vi "HFRR ADV v01.vi"() -> ()   [LabVIEW 2023] (continued)
                n1196 = local write "OK Button 16"(FALSE ("Print 3")) -> ()
              }
            }
          }
        }
        n1197 = case shown="True" "OK Button 17" {
          frame False {
          }
          frame True {
            (unwired) 0  # existing file
            w2745 = "Choose a datalog file to open"  # prompt
            n1198 = local read "String"() -> (w2740:string)
            n1199 = local write "OK Button 17"(FALSE ("OK Button 17")) -> ()
            n1200 = String To Path(string=w2740) -> (path=w2741:path)
            n1201 = File Dialog(6:"*.duf" ("pattern"), 7:w2745, 11:w2741) -> (0:w2732:errorcluster, 3:w2751:path)  [unwired: 4 in, 2 out]
            n1202 = Unbundle(w2732) -> ()  [unwired: 3 out]
            n1203 = Open/Create/Replace File "Open File"(file path (use dialog)=w2751) -> (refnum out=w2743:refnum<file>)  [unwired: 5 in, 2 out]
            n1204 = Path To String(path=w2751) -> (string=w2734:string)
            n1205 = while {
              tunnel: w2743 -> [w2755]
              i -> [w2752]
              stop <- w2753 continue-if-true
              (unwired) TRUE ("line mode (F)")
              n1206 = local write "Numeric 16"(w2752) -> ()
              n1207 = Read from Text File "Read File"(file (use dialog)=w2755) -> (text=w2754:string)  [unwired: 3 in, 3 out]
              n1208 = String Length(string=w2754) -> (length=w2757:i32)
              n1209 = Greater?(x=w2757, y=1) -> (0:w2753:bool)
            }
            n1210 = local write "String 29"(w2734) -> ()
            n1211 = Match Pattern(string=w2734, regular expression=".dwm" ("substring (\"\")")) -> (before substring=w2735:string)  [unwired: 1 in, 3 out]
            "String Indicator 3" <- w2735
            n1212 = Search and Replace String(input string=w2734, search string=".duf", replace string=".dgf" ("replace string (\"\")")) -> (result string=→"String Indicator 4":string)  [unwired: 5 in, 3 out]
            n1213 = String To Path(string=w2735) -> (path=w2742:path)
            "path" <- w2742
            n1214 = Strip Path(path=w2751) -> (name=w2749:string)  [unwired: 1 out]
            n1215 = call <vilib>:"Read Characters From File.vi"("file path (dialog if empty)"=w2742, "start of read offset (chars.:0)"=60 ("start of read offset (chars.: 0)")) -> ("character string"=→"String Indicator 2":string)  [unwired: 4 in, 3 out]
            n1216 = Match Pattern(string=w2749, regular expression=".dwm") -> (before substring=w2733:string)  [unwired: 1 in, 3 out]
            "String Indicator" <- w2733
            n1217 = local write "TITTLE 2"(w2733) -> ()
          }
        }
      }
    }
    n1218 = local read "OK Button 16"() -> (w788:bool)
    n1219 = Or(x=w788, y="OPEN") -> (x .or. y?=w789:bool)
    n1220 = case shown="True" w789 {
      tunnel: w788 -> [_ w841]
      frame False {
      }
      frame True {
        n1221 = stacked-sequence {
          tunnel: w841 -> [_ w908 _ _]
          frame #0 {
            w857 = "  " ("String 6")
            n1222 = local write "OPEN"(FALSE ("open")) -> ()
            n1223 = property on="OPEN" class="Bool (strict)"("Visible"=FALSE) -> ()  [unwired: 2 in, 2 out]
            n1224 = local write "String 12"(w857) -> ()
            n1225 = local write "String 6"(w857) -> ()
            n1226 = local write "String 7"(w857) -> ()
            n1227 = local write "String 8"(w857) -> ()
            n1228 = local read "OK Button 16"() -> (w842:bool)
            n1229 = case shown="True" w842 {
              tunnel: [w858 w859] -> w846
              frame False {
                n1230 = local read "string1"() -> (w858:string)
              }
              frame True {
                n1231 = local read "String Indicator 4"() -> (w859:string)
              }
            }
            n1232 = local read "string1 2"() -> (w845:string)
            n1233 = local read "string1 4"() -> (w843:string)
            n1234 = local read "string1 3"() -> (w844:string)
            n1235 = String To Path(string=w846) -> (path=w854:path)
            n1236 = String To Path(string=w845) -> (path=w853:path)
            n1237 = String To Path(string=w844) -> (path=w852:path)
            n1238 = String To Path(string=w843) -> (path=w851:path)
            n1239 = Open/Create/Replace File "Open File"(file path (use dialog)=w854) -> (refnum out=w850:refnum<file>)  [unwired: 5 in, 2 out]
            n1240 = Open/Create/Replace File "Open File"(file path (use dialog)=w853) -> (refnum out=w849:refnum<file>)  [unwired: 5 in, 2 out]
            n1241 = Open/Create/Replace File "Open File"(file path (use dialog)=w852) -> (refnum out=w848:refnum<file>)  [unwired: 5 in, 2 out]
            n1242 = Open/Create/Replace File "Open File"(file path (use dialog)=w851) -> (refnum out=w847:refnum<file>)  [unwired: 5 in, 2 out]
            n1243 = while {
              tunnel: w850 -> [w865]
              i -> [w861]
              stop <- w860 continue-if-true
              (unwired) TRUE ("line mode (F)")
              n1244 = Read from Text File "Read File"(file (use dialog)=w865) -> (text=w862:string)  [unwired: 3 in, 3 out]
              n1245 = local write "Numeric 8"(w861) -> ()
              n1246 = String Length(string=w862) -> (length=w864:i32)
              n1247 = Greater?(x=w864, y=1) -> (0:w860:bool)
            }
            n1248 = while {
              tunnel: w849 -> [w871]
              i -> [w867]
              stop <- w866 continue-if-true
              (unwired) TRUE ("line mode (F)")
              n1249 = Read from Text File "Read File"(file (use dialog)=w871) -> (text=w868:string)  [unwired: 3 in, 3 out]
              n1250 = local write "Numeric 11"(w867) -> ()
              n1251 = String Length(string=w868) -> (length=w870:i32)
              n1252 = Greater?(x=w870, y=1) -> (0:w866:bool)
            }
            n1253 = while {
              tunnel: w848 -> [w877]
              i -> [w873]
              stop <- w872 continue-if-true
              (unwired) TRUE ("line mode (F)")
              n1254 = Read from Text File "Read File"(file (use dialog)=w877) -> (text=w874:string)  [unwired: 3 in, 3 out]
              n1255 = local write "Numeric 12"(w873) -> ()
              n1256 = String Length(string=w874) -> (length=w876:i32)
              n1257 = Greater?(x=w876, y=1) -> (0:w872:bool)
            }
            n1258 = while {
              tunnel: w847 -> [w883]
              i -> [w879]
              stop <- w878 continue-if-true
              (unwired) TRUE ("line mode (F)")
              n1259 = Read from Text File "Read File"(file (use dialog)=w883) -> (text=w880:string)  [unwired: 3 in, 3 out]
              n1260 = local write "Numeric 13"(w879) -> ()
              n1261 = String Length(string=w880) -> (length=w882:i32)
              n1262 = Greater?(x=w882, y=1) -> (0:w878:bool)
            }
          }
          frame #1 {
            w1035 = FALSE ("ACTUAL   MERGE")
            # "Sample Temp"
            # "ECR"
            # "COF"
            # "Time\nCOF\nFF\nTemp"
            n1263 = case shown="True" w908 {
              tunnel: [w1055 w1056] -> w909
              frame False {
                n1264 = local read "string1"() -> (w1055:string)
              }
              frame True {
                n1265 = local read "String Indicator 4"() -> (w1056:string)
              }
            }
            n1266 = local read "string1 2"() -> (w954:string)
            n1267 = local read "string1 4"() -> (w952:string)
            n1268 = local read "string1 3"() -> (w953:string)
            n1269 = String To Path(string=w952) -> (path=w1046:path)
            n1270 = String To Path(string=w954) -> (path=w1052:path)
            n1271 = String To Path(string=w909) -> (path=w1040:path)
            n1272 = Open/Create/Replace File "Open File"(file path (use dialog)=w1046) -> (refnum out=w1045:refnum<file>, error out=w1044:errorcluster)  [unwired: 5 in, 1 out]
            n1273 = Open/Create/Replace File "Open File"(file path (use dialog)=w1040) -> (refnum out=w1054:refnum<file>, error out=w1053:errorcluster)  [unwired: 5 in, 1 out]
            n1274 = Open/Create/Replace File "Open File"(file path (use dialog)=w1052) -> (refnum out=w1050:refnum<file>, error out=w1049:errorcluster)  [unwired: 5 in, 1 out]
            n1275 = String To Path(string=w953) -> (path=w1051:path)
            n1276 = local read "Numeric 8"() -> (w1039:i32)
            n1277 = Open/Create/Replace File "Open File"(file path (use dialog)=w1051) -> (refnum out=w1047:refnum<file>, error out=w1048:errorcluster)  [unwired: 5 in, 1 out]
            n1278 = local read "Numeric 13"() -> (w1038:i32)
            n1279 = local read "Numeric 11"() -> (w1036:i32)
            n1280 = local read "Numeric 12"() -> (w1037:i32)
            n1281 = for {
              N: w1036 -> [_]
              tunnel: w1050 -> [w1165]
              tunnel: w1049 -> [w1164]
              tunnel: [w1154] -> w1016 mode=indexing
              tunnel: [w1152] -> w1014 mode=indexing
              tunnel: [w1153] -> w1009 mode=indexing
              tunnel: w1035 -> [_]
              tunnel: [w1146] -> w1011 mode=indexing
              tunnel: [w1142] -> w987 mode=indexing
              tunnel: [w1138] -> w962 mode=indexing
              tunnel: [w1134] -> w943 mode=indexing
              tunnel: [w1129] -> w901 mode=indexing
              (unwired) TRUE ("line mode (F)")
              n1282 = Read from Text File "Read File"(file (use dialog)=w1165, error in=w1164) -> (text=w1130:string)  [unwired: 2 in, 3 out]
              n1283 = String Subset(string=w1130, offset (0)=0, length (rest)=14 ("length (rest)")) -> (substring=w1158:string)
              n1284 = Fract/Exp String To Number(string=w1158) -> (number=w1154:dbl)  [unwired: 3 in, 1 out]
              n1285 = local write "String 7"(w1130) -> ()
              n1286 = String Subset(string=w1130, offset (0)=15, length (rest)=9 ("length (rest)")) -> (substring=w1161:string)
              n1287 = Fract/Exp String To Number(string=w1161) -> (number=w1152:dbl)  [unwired: 3 in, 1 out]
              n1288 = String Subset(string=w1130, offset (0)=65, length (rest)=9 ("length (rest)")) -> (substring=w1147:string)
              n1289 = Fract/Exp String To Number(string=w1147) -> (number=w1150:dbl)  [unwired: 3 in, 1 out]
              n1290 = Add(x=w1150, y=0.0) -> (x+y=w1146:dbl)
              n1291 = String Subset(string=w1130, offset (0)=35, length (rest)=9 ("length (rest)")) -> (substring=w1155:string)
              n1292 = Fract/Exp String To Number(string=w1155) -> (number=w1153:dbl)  [unwired: 3 in, 1 out]
              n1293 = String Subset(string=w1130, offset (0)=45, length (rest)=9 ("length (rest)")) -> (substring=w1143:string)
              n1294 = Fract/Exp String To Number(string=w1143) -> (number=w1142:dbl)  [unwired: 3 in, 1 out]
              n1295 = String Subset(string=w1130, offset (0)=55, length (rest)=9 ("length (rest)")) -> (substring=w1141:string)
              n1296 = Fract/Exp String To Number(string=w1141) -> (number=w1138:dbl)  [unwired: 3 in, 1 out]
              n1297 = String Subset(string=w1130, offset (0)=25, length (rest)=9 ("length (rest)")) -> (substring=w1135:string)
              n1298 = Fract/Exp String To Number(string=w1135) -> (number=w1134:dbl)  [unwired: 3 in, 1 out]
              n1299 = String Subset(string=w1130, offset (0)=85, length (rest)=9 ("length (rest)")) -> (substring=w1133:string)
              n1300 = Fract/Exp String To Number(string=w1133) -> (number=w1129:dbl)  [unwired: 3 in, 1 out]
            }
            n1301 = for {
              N: w1037 -> [_]
              tunnel: w1048 -> [w1128]
              tunnel: w1047 -> [w1127]
              tunnel: [w1117] -> w1006 mode=indexing
              tunnel: [w1115] -> w1004 mode=indexing
              tunnel: [w1116] -> w1000 mode=indexing
              tunnel: w1035 -> [_]
              tunnel: [w1109] -> w1002 mode=indexing
              tunnel: [w1105] -> w984 mode=indexing
              tunnel: [w1101] -> w960 mode=indexing
              tunnel: [w1098] -> w941 mode=indexing
              tunnel: [w1094] -> w900 mode=indexing
              (unwired) 9 ("length (rest)")
              (unwired) 9 ("length (rest)")
              (unwired) TRUE ("line mode (F)")
              n1302 = Read from Text File "Read File"(file (use dialog)=w1127, error in=w1128) -> (text=w1095:string)  [unwired: 2 in, 3 out]
              n1303 = String Subset(string=w1095, offset (0)=0, length (rest)=14 ("length (rest)")) -> (substring=w1121:string)
              n1304 = Fract/Exp String To Number(string=w1121) -> (number=w1117:dbl)  [unwired: 3 in, 1 out]
              n1305 = local write "String 8"(w1095) -> ()
              n1306 = String Subset(string=w1095, offset (0)=15, length (rest)=9 ("length (rest)")) -> (substring=w1124:string)
              n1307 = Fract/Exp String To Number(string=w1124) -> (number=w1115:dbl)  [unwired: 3 in, 1 out]
              n1308 = String Subset(string=w1095, offset (0)=65, length (rest)=9 ("length (rest)")) -> (substring=w1114:string)
              n1309 = Fract/Exp String To Number(string=w1114) -> (number=w1111:dbl)  [unwired: 3 in, 1 out]
              n1310 = Add(x=w1111, y=0.0) -> (x+y=w1109:dbl)
              n1311 = String Subset(string=w1095, offset (0)=35, length (rest)=9 ("length (rest)")) -> (substring=w1118:string)
              n1312 = Fract/Exp String To Number(string=w1118) -> (number=w1116:dbl)  [unwired: 3 in, 1 out]
              n1313 = String Subset(string=w1095, offset (0)=45, length (rest)=9 ("length (rest)")) -> (substring=w1108:string)
              n1314 = Fract/Exp String To Number(string=w1108) -> (number=w1105:dbl)  [unwired: 3 in, 1 out]
              n1315 = String Subset(string=w1095, offset (0)=55, length (rest)=9 ("length (rest)")) -> (substring=w1103:string)
              n1316 = Fract/Exp String To Number(string=w1103) -> (number=w1101:dbl)  [unwired: 3 in, 1 out]
              n1317 = String Subset(string=w1095, offset (0)=25) -> (substring=w1099:string)  [unwired: 1 in]
              n1318 = Fract/Exp String To Number(string=w1099) -> (number=w1098:dbl)  [unwired: 3 in, 1 out]
              n1319 = String Subset(string=w1095, offset (0)=85) -> (substring=w1097:string)  [unwired: 1 in]
              n1320 = Fract/Exp String To Number(string=w1097) -> (number=w1094:dbl)  [unwired: 3 in, 1 out]
            }
            n1321 = for {
              N: w1038 -> [_]
              tunnel: w1045 -> [w1093]
              tunnel: w1044 -> [w1092]
              tunnel: [w1082] -> w998 mode=indexing
              tunnel: [w1081] -> w991 mode=indexing
              tunnel: w1035 -> [_]
              tunnel: [w1070] -> w996 mode=indexing
              tunnel: [w1075] -> w993 mode=indexing
              tunnel: [w1071] -> w983 mode=indexing
              tunnel: [w1066] -> w958 mode=indexing
              tunnel: [w1062] -> w939 mode=indexing
              tunnel: [w1057] -> w899 mode=indexing
              (unwired) 1.0 ("x")
              (unwired) TRUE ("line mode (F)")
              n1322 = Read from Text File "Read File"(file (use dialog)=w1093, error in=w1092) -> (text=w1058:string)  [unwired: 2 in, 3 out]
              n1323 = String Subset(string=w1058, offset (0)=0, length (rest)=14 ("length (rest)")) -> (substring=w1086:string)
              n1324 = Fract/Exp String To Number(string=w1086) -> (number=w1082:dbl)  [unwired: 3 in, 1 out]
              n1325 = String Subset(string=w1058, offset (0)=15, length (rest)=9 ("length (rest)")) -> (substring=w1089:string)
              n1326 = local write "String 12"(w1058) -> ()
              n1327 = Fract/Exp String To Number(string=w1089) -> (number=w1070:dbl)  [unwired: 3 in, 1 out]
              n1328 = String Subset(string=w1058, offset (0)=65, length (rest)=9 ("length (rest)")) -> (substring=w1076:string)
              n1329 = Fract/Exp String To Number(string=w1076) -> (number=w1079:dbl)  [unwired: 3 in, 1 out]
              n1330 = Add(x=w1079, y=0.0) -> (x+y=w1075:dbl)
              n1331 = String Subset(string=w1058, offset (0)=35, length (rest)=9 ("length (rest)")) -> (substring=w1083:string)
              n1332 = Fract/Exp String To Number(string=w1083) -> (number=w1081:dbl)  [unwired: 3 in, 1 out]
              n1333 = String Subset(string=w1058, offset (0)=45, length (rest)=9 ("length (rest)")) -> (substring=w1073:string)
              n1334 = Fract/Exp String To Number(string=w1073) -> (number=w1071:dbl)  [unwired: 3 in, 1 out]
              n1335 = String Subset(string=w1058, offset (0)=55, length (rest)=9 ("length (rest)")) -> (substring=w1068:string)
              n1336 = Fract/Exp String To Number(string=w1068) -> (number=w1066:dbl)  [unwired: 3 in, 1 out]
              n1337 = String Subset(string=w1058, offset (0)=25, length (rest)=9 ("length (rest)")) -> (substring=w1064:string)
              n1338 = Fract/Exp String To Number(string=w1064) -> (number=w1062:dbl)  [unwired: 3 in, 1 out]
              n1339 = String Subset(string=w1058, offset (0)=85, length (rest)=9 ("length (rest)")) -> (substring=w1060:string)
              n1340 = Fract/Exp String To Number(string=w1060) -> (number=w1057:dbl)  [unwired: 3 in, 1 out]
            }
            n1341 = for {
              N: w1039 -> [_]
              tunnel: w1054 -> [w1202]
              tunnel: w1053 -> [w1201]
              tunnel: [w1191] -> w966 mode=indexing
              tunnel: [w1189] -> w1023 mode=indexing
              tunnel: [w1190] -> w1018 mode=indexing
              tunnel: w1035 -> [_]
              tunnel: [w1183] -> w1020 mode=indexing
              tunnel: [w1179] -> w989 mode=indexing
              tunnel: [w1175] -> w964 mode=indexing
              tunnel: [w1171] -> w945 mode=indexing
              tunnel: [w1166] -> w905 mode=indexing
              (unwired) TRUE ("line mode (F)")
              # "freq"
              # "Stroke"
              # "Time"
              # "CoF"
              # "Humidity"
              # "Temp"
              # "Air Temp"
              # "ECR"
              n1342 = Read from Text File "Read File"(file (use dialog)=w1202, error in=w1201) -> (text=w1167:string)  [unwired: 2 in, 3 out]
              n1343 = String Subset(string=w1167, offset (0)=0, length (rest)=14 ("length (rest)")) -> (substring=w1195:string)
              n1344 = Fract/Exp String To Number(string=w1195) -> (number=w1191:dbl)  [unwired: 3 in, 1 out]
              n1345 = local write "String 6"(w1167) -> ()
              n1346 = String Subset(string=w1167, offset (0)=15, length (rest)=9 ("length (rest)")) -> (substring=w1198:string)
              n1347 = Fract/Exp String To Number(string=w1198) -> (number=w1189:dbl)  [unwired: 3 in, 1 out]
              n1348 = String Subset(string=w1167, offset (0)=65, length (rest)=9 ("length (rest)")) -> (substring=w1188:string)
              n1349 = Fract/Exp String To Number(string=w1188) -> (number=w1185:dbl)  [unwired: 3 in, 1 out]
              n1350 = Add(x=w1185, y=0.0) -> (x+y=w1183:dbl)
              n1351 = String Subset(string=w1167, offset (0)=35, length (rest)=9 ("length (rest)")) -> (substring=w1192:string)
              n1352 = Fract/Exp String To Number(string=w1192) -> (number=w1190:dbl)  [unwired: 3 in, 1 out]
              n1353 = String Subset(string=w1167, offset (0)=45, length (rest)=9 ("length (rest)")) -> (substring=w1182:string)
              n1354 = Fract/Exp String To Number(string=w1182) -> (number=w1179:dbl)  [unwired: 3 in, 1 out]
              n1355 = String Subset(string=w1167, offset (0)=55, length (rest)=9 ("length (rest)")) -> (substring=w1176:string)
              n1356 = Fract/Exp String To Number(string=w1176) -> (number=w1175:dbl)  [unwired: 3 in, 1 out]
              n1357 = String Subset(string=w1167, offset (0)=25, length (rest)=9 ("length (rest)")) -> (substring=w1174:string)
              n1358 = Fract/Exp String To Number(string=w1174) -> (number=w1171:dbl)  [unwired: 3 in, 1 out]
              n1359 = String Subset(string=w1167, offset (0)=85, length (rest)=9 ("length (rest)")) -> (substring=w1168:string)
              n1360 = Fract/Exp String To Number(string=w1168) -> (number=w1166:dbl)  [unwired: 3 in, 1 out]
            }
            n1361 = Delete From Array(array=w1006, index=0) -> (array with subset deleted=w889:dbl[])  [unwired: 1 in, 1 out]
            n1362 = Delete From Array(array=w998, index=0) -> (array with subset deleted=w887:dbl[])  [unwired: 1 in, 1 out]
            n1363 = Delete From Array(array=w1016, index=0) -> (array with subset deleted=w891:dbl[])  [unwired: 1 in, 1 out]
            n1364 = Delete From Array(array=w996, index=0) -> (array with subset deleted=w976:dbl[])  [unwired: 1 in, 1 out]
            n1365 = Delete From Array(array=w966, index=0) -> (array with subset deleted=w893:dbl[])  [unwired: 1 in, 1 out]
            n1366 = Delete From Array(array=w1004, index=0) -> (array with subset deleted=w977:dbl[])  [unwired: 1 in, 1 out]
            n1367 = Delete From Array(array=w1014, index=0) -> (array with subset deleted=w975:dbl[])  [unwired: 1 in, 1 out]
            n1368 = Delete From Array(array=w1023, index=0) -> (array with subset deleted=w978:dbl[])  [unwired: 1 in, 1 out]
            n1369 = Bundle "Bundle"(w887, w976) -> (w1041:cluster{dbl[], dbl[]})  [unwired: 1 in]
            n1370 = Bundle "Bundle"(w891, w975) -> (w1043:cluster{dbl[], dbl[]})  [unwired: 1 in]
            n1371 = Bundle "Bundle"(w889, w977) -> (w1042:cluster{dbl[], dbl[]})  [unwired: 1 in]
            n1372 = Bundle "Bundle"(w893, w978) -> (w912:cluster{dbl[], dbl[]})  [unwired: 1 in]
            n1373 = Build Array "Build Array"(w912, w1043, w1042, w1041) -> (→"XY Graph 9":cluster{dbl[], dbl[]}[])
            n1374 = Delete From Array(array=w1011, index=0) -> (array with subset deleted=w1012:dbl[])  [unwired: 1 in, 1 out]
            n1375 = Delete From Array(array=w993, index=0) -> (array with subset deleted=w994:dbl[])  [unwired: 1 in, 1 out]
            n1376 = Delete From Array(array=w1002, index=0) -> (array with subset deleted=w1003:dbl[])  [unwired: 1 in, 1 out]
            n1377 = Delete From Array(array=w1020, index=0) -> (array with subset deleted=w1021:dbl[])  [unwired: 1 in, 1 out]
            n1378 = Delete From Array(array=w991, index=0) -> (array with subset deleted=w921:dbl[])  [unwired: 1 in, 1 out]
            n1379 = Delete From Array(array=w1000, index=0) -> (array with subset deleted=w922:dbl[])  [unwired: 1 in, 1 out]
            n1380 = Delete From Array(array=w1018, index=0) -> (array with subset deleted=w924:dbl[])  [unwired: 1 in, 1 out]
            n1381 = Delete From Array(array=w1009, index=0) -> (array with subset deleted=w923:dbl[])  [unwired: 1 in, 1 out]
            n1382 = Bundle "Bundle"(w887, w921) -> (w1033:cluster{dbl[], dbl[]})  [unwired: 1 in]
            n1383 = Bundle "Bundle"(w891, w923) -> (w1034:cluster{dbl[], dbl[]})  [unwired: 1 in]
            n1384 = Bundle "Bundle"(w889, w922) -> (w1032:cluster{dbl[], dbl[]})  [unwired: 1 in]
            n1385 = Bundle "Bundle"(w893, w924) -> (w911:cluster{dbl[], dbl[]})  [unwired: 1 in]
            n1386 = Delete From Array(array=w984, index=0) -> (array with subset deleted=w972:dbl[])  [unwired: 1 in, 1 out]
            n1387 = Build Array "Build Array"(w911, w1034, w1032, w1033) -> (→"XY Graph 10":cluster{dbl[], dbl[]}[])
            n1388 = Delete From Array(array=w989, index=0) -> (array with subset deleted=w974:dbl[])  [unwired: 1 in, 1 out]
            "array w/ subset deleted" <- w974
            n1389 = Delete From Array(array=w987, index=0) -> (array with subset deleted=w973:dbl[])  [unwired: 1 in, 1 out]
            n1390 = Delete From Array(array=w964, index=0) -> (array with subset deleted=w920:dbl[])  [unwired: 1 in, 1 out]
            n1391 = Bundle "Bundle"(w887, w994) -> (w1026:cluster{dbl[], dbl[]})  [unwired: 1 in]
            n1392 = Bundle "Bundle"(w891, w1012) -> (w1025:cluster{dbl[], dbl[]})  [unwired: 1 in]
            n1393 = Bundle "Bundle"(w889, w1003) -> (w1027:cluster{dbl[], dbl[]})  [unwired: 1 in]
            n1394 = Bundle "Bundle"(w893, w1021) -> (w885:cluster{dbl[], dbl[]})  [unwired: 1 in]
            n1395 = Build Array "Build Array"(w885, w1025, w1027, w1026) -> (→"XY Graph 13":cluster{dbl[], dbl[]}[])
            n1396 = Delete From Array(array=w983, index=0) -> (array with subset deleted=w971:dbl[])  [unwired: 1 in, 1 out]
            n1397 = Delete From Array(array=w958, index=0) -> (array with subset deleted=w917:dbl[])  [unwired: 1 in, 1 out]
            n1398 = Delete From Array(array=w962, index=0) -> (array with subset deleted=w919:dbl[])  [unwired: 1 in, 1 out]
            n1399 = Delete From Array(array=w960, index=0) -> (array with subset deleted=w918:dbl[])  [unwired: 1 in, 1 out]
            n1400 = call-poly <vilib>:"Mean.vi"("X"=w976) -> ("mean"=→"КОФ4":dbl)  [unwired: 1 out]
            n1401 = call-poly <vilib>:"Mean.vi"("X"=w978) -> ("mean"=→"КОФ1":dbl)  [unwired: 1 out]
            n1402 = call-poly <vilib>:"Mean.vi"("X"=w977) -> ("mean"=→"КОФ3":dbl)  [unwired: 1 out]
            n1403 = Bundle "Bundle"(w893, w974) -> (w907:cluster{dbl[], dbl[]})  [unwired: 1 in]
            n1404 = Bundle "Bundle"(w887, w971) -> (w979:cluster{dbl[], dbl[]})  [unwired: 1 in]
            n1405 = Bundle "Bundle"(w891, w973) -> (w981:cluster{dbl[], dbl[]})  [unwired: 1 in]
            n1406 = Bundle "Bundle"(w889, w972) -> (w980:cluster{dbl[], dbl[]})  [unwired: 1 in]
            n1407 = call-poly <vilib>:"Mean.vi"("X"=w975) -> ("mean"=→"КОФ2":dbl)  [unwired: 1 out]
            n1408 = Build Array "Build Array"(w907, w981, w980, w979) -> (→"XY Graph 12":cluster{dbl[], dbl[]}[])
            n1409 = Bundle "Bundle"(w893, w920) -> (w884:cluster{dbl[], dbl[]})  [unwired: 1 in]
            n1410 = Bundle "Bundle"(w887, w917) -> (w955:cluster{dbl[], dbl[]})  [unwired: 1 in]
            n1411 = Bundle "Bundle"(w891, w919) -> (w957:cluster{dbl[], dbl[]})  [unwired: 1 in]
            n1412 = Bundle "Bundle"(w889, w918) -> (w956:cluster{dbl[], dbl[]})  [unwired: 1 in]
            n1413 = Delete From Array(array=w943, index=0) -> (array with subset deleted=w915:dbl[])  [unwired: 1 in, 1 out]
            n1414 = Delete From Array(array=w941, index=0) -> (array with subset deleted=w914:dbl[])  [unwired: 1 in, 1 out]
            n1415 = call-poly <vilib>:"Mean.vi"("X"=w973) -> ("mean"=→"CP2":dbl)  [unwired: 1 out]
            n1416 = call-poly <vilib>:"Mean.vi"("X"=w971) -> ("mean"=→"CP4":dbl)  [unwired: 1 out]
            n1417 = Build Array "Build Array"(w884, w957, w956, w955) -> (→"XY Graph 11":cluster{dbl[], dbl[]}[])
            n1418 = call-poly <vilib>:"Mean.vi"("X"=w972) -> ("mean"=→"CP3":dbl)  [unwired: 1 out]
            n1419 = call-poly <vilib>:"Mean.vi"("X"=w974) -> ("mean"=→"CP1":dbl)  [unwired: 1 out]
            n1420 = Delete From Array(array=w945, index=0) -> (array with subset deleted=w916:dbl[])  [unwired: 1 in, 1 out]
            n1421 = Bundle "Bundle"(w924, w920) -> (w926:cluster{dbl[], dbl[]})  [unwired: 1 in]
            n1422 = Bundle "Bundle"(w921, w917) -> (w929:cluster{dbl[], dbl[]})  [unwired: 1 in]
            n1423 = Bundle "Bundle"(w923, w919) -> (w927:cluster{dbl[], dbl[]})  [unwired: 1 in]
            n1424 = Bundle "Bundle"(w922, w918) -> (w928:cluster{dbl[], dbl[]})  [unwired: 1 in]
            n1425 = Delete From Array(array=w939, index=0) -> (array with subset deleted=w913:dbl[])  [unwired: 1 in, 1 out]
            n1426 = Build Array "Build Array"(w926, w927, w928, w929) -> (→"XY Graph 15":cluster{dbl[], dbl[]}[])
            n1427 = Build Array "Build Array"(w884, w907) -> (w910:cluster{dbl[], dbl[]}[])
            "XY Graph 17" <- w910
            n1428 = local write "XY Graph 16"(w910) -> ()
            n1429 = Bundle "Bundle"(w891, w915) -> (w937:cluster{dbl[], dbl[]})  [unwired: 1 in]
            n1430 = Bundle "Bundle"(w889, w914) -> (w936:cluster{dbl[], dbl[]})  [unwired: 1 in]
            n1431 = Bundle "Bundle"(w887, w913) -> (w935:cluster{dbl[], dbl[]})  [unwired: 1 in]
            n1432 = Bundle "Bundle"(w893, w916) -> (w938:cluster{dbl[], dbl[]})  [unwired: 1 in]
            n1433 = Delete From Array(array=w905, index=0) -> (array with subset deleted=w892:dbl[])  [unwired: 1 in, 1 out]
            n1434 = Delete From Array(array=w901, index=0) -> (array with subset deleted=w890:dbl[])  [unwired: 1 in, 1 out]
            n1435 = Build Array "Build Array"(w938, w937, w936, w935) -> (→"XY Graph 14":cluster{dbl[], dbl[]}[])
            n1436 = Delete From Array(array=w899, index=0) -> (array with subset deleted=w886:dbl[])  [unwired: 1 in, 1 out]
            n1437 = Delete From Array(array=w900, index=0) -> (array with subset deleted=w888:dbl[])  [unwired: 1 in, 1 out]
            n1438 = Bundle "Bundle"(w893, w892) -> (w898:cluster{dbl[], dbl[]})  [unwired: 1 in]
            n1439 = Bundle "Bundle"(w891, w890) -> (w897:cluster{dbl[], dbl[]})  [unwired: 1 in]
            n1440 = call-poly <vilib>:"Mean.vi"("X"=w916) -> ("mean"=→"КОФ2 2":dbl)  [unwired: 1 out]
            n1441 = Bundle "Bundle"(w887, w886) -> (w895:cluster{dbl[], dbl[]})  [unwired: 1 in]
            n1442 = Bundle "Bundle"(w889, w888) -> (w896:cluster{dbl[], dbl[]})  [unwired: 1 in]
            n1443 = call-poly <vilib>:"Mean.vi"("X"=w915) -> ("mean"=→"КОФ2 3":dbl)  [unwired: 1 out]
            n1444 = call-poly <vilib>:"Mean.vi"("X"=w913) -> ("mean"=→"КОФ2 5":dbl)  [unwired: 1 out]
            n1445 = call-poly <vilib>:"Mean.vi"("X"=w914) -> ("mean"=→"КОФ2 4":dbl)  [unwired: 1 out]
            n1446 = Build Array "Build Array"(w898, w897, w896, w895) -> (→"XY Graph 18":cluster{dbl[], dbl[]}[])
          }
          frame #2 {
          }
          frame #3 {
            n1447 = local read "String Control 4"() -> (w1209:string)
            n1448 = local read "String Control 6"() -> (w1208:string)
            n1449 = local read "String Control 8"() -> (w1207:string)
            n1450 = local read "String Control 2"() -> (w1210:string)
            n1451 = property on="OPEN" class="Bool (strict)"("Visible"=TRUE) -> ()  [unwired: 2 in, 2 out]
            n1452 = Match Pattern(string=w1208, regular expression="Frequency :- ") -> (after substring=w1233:string)  [unwired: 1 in, 3 out]
            n1453 = Match Pattern(string=w1210, regular expression="Frequency :- ") -> (after substring=w1243:string)  [unwired: 1 in, 3 out]
            n1454 = Match Pattern(string=w1209, regular expression="Frequency :- ") -> (after substring=w1238:string)  [unwired: 1 in, 3 out]
            n1455 = Match Pattern(string=w1207, regular expression="Frequency :- ") -> (after substring=w1228:string)  [unwired: 1 in, 3 out]
            n1456 = String Subset(string=w1233, length (rest)=9 ("length (rest)")) -> (substring=w1235:string)  [unwired: 1 in]
            n1457 = String Subset(string=w1243, length (rest)=9 ("length (rest)")) -> (substring=w1245:string)  [unwired: 1 in]
            n1458 = String Subset(string=w1238, length (rest)=9 ("length (rest)")) -> (substring=w1240:string)  [unwired: 1 in]
            n1459 = String Subset(string=w1228, length (rest)=9 ("length (rest)")) -> (substring=w1230:string)  [unwired: 1 in]
            n1460 = Fract/Exp String To Number(string=w1235) -> (number=w1236:dbl)  [unwired: 3 in, 1 out]
            n1461 = Fract/Exp String To Number(string=w1245) -> (number=w1246:dbl)  [unwired: 3 in, 1 out]
            n1462 = Fract/Exp String To Number(string=w1240) -> (number=w1241:dbl)  [unwired: 3 in, 1 out]
            n1463 = Fract/Exp String To Number(string=w1230) -> (number=w1231:dbl)  [unwired: 3 in, 1 out]
            n1464 = local write "freq3"(w1236) -> ()
            n1465 = local write "freq2"(w1241) -> ()
            n1466 = local write "freq1"(w1246) -> ()
            n1467 = local write "freq 4"(w1231) -> ()
            n1468 = local write "Numeric 13"(0 ("Numeric 13")) -> ()
            n1469 = local write "Numeric 11"(0 ("Numeric 11")) -> ()
            n1470 = local write "Numeric 8"(0 ("Numeric 8")) -> ()
            n1471 = local write "Numeric 12"(0 ("Numeric 12")) -> ()
            n1472 = Match Pattern(string=w1208, regular expression="Samples / cycle :- ") -> (after substring=w1216:string)  [unwired: 1 in, 3 out]
            n1473 = Match Pattern(string=w1210, regular expression="Samples / cycle :- ") -> (after substring=w1224:string)  [unwired: 1 in, 3 out]
            n1474 = Match Pattern(string=w1209, regular expression="Samples / cycle :- ") -> (after substring=w1220:string)  [unwired: 1 in, 3 out]
            n1475 = Match Pattern(string=w1207, regular expression="Samples / cycle :- ") -> (after substring=w1212:string)  [unwired: 1 in, 3 out]
            n1476 = String Subset(string=w1216, length (rest)=6 ("length (rest)")) -> (substring=w1218:string)  [unwired: 1 in]
            n1477 = String Subset(string=w1224, length (rest)=6 ("length (rest)")) -> (substring=w1226:string)  [unwired: 1 in]
            n1478 = String Subset(string=w1220, length (rest)=6 ("length (rest)")) -> (substring=w1222:string)  [unwired: 1 in]
            n1479 = String Subset(string=w1212, length (rest)=6 ("length (rest)")) -> (substring=w1214:string)  [unwired: 1 in]
            n1480 = Fract/Exp String To Number(string=w1218) -> (number=w1204:dbl)  [unwired: 3 in, 1 out]
            n1481 = Fract/Exp String To Number(string=w1226) -> (number=w1206:dbl)  [unwired: 3 in, 1 out]
            n1482 = Fract/Exp String To Number(string=w1222) -> (number=w1205:dbl)  [unwired: 3 in, 1 out]
            n1483 = Fract/Exp String To Number(string=w1214) -> (number=w1203:dbl)  [unwired: 3 in, 1 out]
            n1484 = local write "sample2"(w1205) -> ()
            n1485 = local write "sample3"(w1204) -> ()
            n1486 = local write "sample1"(w1206) -> ()
            n1487 = local write "sample4"(w1203) -> ()
          }
        }
      }
    }
    n1488 = Wait (ms)(milliseconds to wait=u32 50) -> ()  [unwired: 1 out]
    n1489 = property on="STOP 3" class="Bool (strict)"() -> ("Visible"=w800:bool)  [unwired: 2 in, 2 out]
    n1490 = case shown="True" w800 {
      frame False {
      }
      frame True {
        n1491 = case shown="True" "Save Results" {
          frame False {
          }
          frame True {
            w1732 = "\r"
            n1492 = local read "Temperature before test"() -> (w1770:dbl)
            n1493 = local read "Temperature after test"() -> (w1772:dbl)
            n1494 = local read "Humidity before test"() -> (w1769:dbl)
            n1495 = local read "Humidity after test"() -> (w1771:dbl)
            n1496 = local read "MWSD"() -> (w1773:dbl)
            n1497 = local read "WS1.4"() -> (w1776:dbl)
            n1498 = local read "AVP"() -> (w1774:dbl)
            n1499 = local read "HCF"() -> (w1775:dbl)
            n1500 = local write "Save Results"(FALSE ("OK Button 5")) -> ()
            n1501 = Number To Fractional String(number=w1772, width (-)=i16 6, precision (6)=i16 1) -> (F-format string=w1750:string)  [unwired: 1 in]
            n1502 = Number To Fractional String(number=w1773, width (-)=i16 6, precision (6)=i16 1) -> (F-format string=w1747:string)  [unwired: 1 in]
            n1503 = Number To Fractional String(number=w1774, width (-)=i16 6, precision (6)=i16 3) -> (F-format string=w1743:string)  [unwired: 1 in]
            n1504 = Number To Fractional String(number=w1771, width (-)=i16 6, precision (6)=i16 1) -> (F-format string=w1754:string)  [unwired: 1 in]
            n1505 = Number To Fractional String(number=w1775, width (-)=i16 6, precision (6)=i16 2) -> (F-format string=w1741:string)  [unwired: 1 in]
            n1506 = Number To Fractional String(number=w1776, width (-)=i16 6, precision (6)=i16 1) -> (F-format string=w1736:string)  [unwired: 1 in]
            n1507 = Number To Fractional String(number=w1770, width (-)=i16 6, precision (6)=i16 1) -> (F-format string=w1758:string)  [unwired: 1 in]
            n1508 = Number To Fractional String(number=w1769, width (-)=i16 6, precision (6)=i16 1) -> (F-format string=w1761:string)  [unwired: 1 in]
            n1509 = local read "String"() -> (w1765:string)
            n1510 = local read "FILE"() -> (w1768:string)
            n1511 = Concatenate Strings(w1765, w1768) -> (w1787:string)
            n1512 = Concatenate Strings(w1787, ".dwm" ("Substring")) -> (w1785:string)
            n1513 = Concatenate Strings(w1741, ")" ("string")) -> (w1739:string)
            n1514 = Concatenate Strings("(" ("string"), w1736, ")Microns" ("string")) -> (w1735:string)
            n1515 = Concatenate Strings("(" ("string"), w1761, " ) % RH," ("string")) -> (w1762:string)
            n1516 = Concatenate Strings("(" ("string"), w1743, ")  kPa," ("string")) -> (w1733:string)
            n1517 = String To Path(string=w1785) -> (path=w1784:path)
            n1518 = Concatenate Strings("(" ("string"), w1758, ")  Deg C ," ("string")) -> (w1757:string)
            n1519 = Concatenate Strings("(" ("string"), w1754, " ) % RH," ("string")) -> (w1753:string)
            n1520 = Concatenate Strings("(" ("string"), w1750, ")  Deg C ," ("string")) -> (w1749:string)
            n1521 = Concatenate Strings("(" ("string"), w1747, ")  Microns," ("string")) -> (w1746:string)
            n1522 = local read "REMARKS"() -> (w1767:string)
            "REMARKS 2" <- w1767
            n1523 = Concatenate Strings(w1767, w1732, " Humidity before test= " ("Substring"), w1762, w1732, " Temperature before test = " ("Substring"), w1757, w1732, " Humidity after test= " ("Substring"), w1753, w1732, "Temperature after test = " ("Substring"), w1749, w1732, "MSD = " ("Substring"), w1746, w1732, "  AVP = " ("Substring"), w1733, w1732, "  HCF                     =( " ("Substring"), w1739, w1732, " WS1.4                  = " ("Substring"), w1735, w1732) -> (w1731:string)
            "data" <- w1731
            n1524 = call <vilib>:"Write Characters To File.vi"("append to file? (new file:F)"=FALSE, "character string"=w1731, "file path (dialog if empty)"=w1784) -> ()  [unwired: 2 in, 1 out]
            n1525 = Match Pattern(string=w1731, regular expression="!") -> (after substring=→"export":string)  [unwired: 1 in, 3 out]
          }
        }
        n1526 = local read "Temperature before test"() -> (w1700:dbl)
        n1527 = local read "Humidity before test"() -> (w1702:dbl)
        n1528 = local read "Temperature after test"() -> (w1716:dbl)
        n1529 = Add(x=231.864, y=w1700) -> (x+y=w1697:dbl)
        n1530 = Add(x=231.864, y=w1716) -> (x+y=w1713:dbl)
        n1531 = local read "Humidity after test"() -> (w1718:dbl)
        n1532 = Divide(x=1705.984, y=w1697) -> (x/y=w1698:dbl)
        n1533 = Divide(x=1705.984, y=w1713) -> (x/y=w1714:dbl)
        n1534 = Subtract(x=8.017352 ("y"), y=w1698) -> (x-y=w1727:dbl)
        n1535 = expression code="10**y"(w1727) -> (w1704:dbl)
        n1536 = Subtract(x=8.017352 ("y"), y=w1714) -> (x-y=w1721:dbl)
        n1537 = expression code="10**y"(w1721) -> (w1720:dbl)
        n1538 = Multiply(x=w1702, y=w1704) -> (x*y=w1703:dbl)
        n1539 = Multiply(x=w1718, y=w1720) -> (x*y=w1719:dbl)
        n1540 = Divide(x=w1703, y=750.0) -> (x/y=w1722:dbl)
        n1541 = Divide(x=w1719, y=750.0) -> (x/y=w1723:dbl)
        n1542 = Add(x=w1722, y=w1723) -> (x+y=w1724:dbl)
        n1543 = Divide(x=w1724, y=2.0) -> (x/y=w1726:dbl)
        n1544 = local write "AVP"(w1726) -> ()
        n1545 = local read "HCF"() -> (w1709:dbl)
        n1546 = Subtract(x=1.4, y=w1726) -> (x-y=w1707:dbl)
        n1547 = local read "MWSD"() -> (w1705:dbl)
        n1548 = Multiply(x=w1707, y=w1709) -> (x*y=w1708:dbl)
        n1549 = Add(x=w1708, y=w1705) -> (x+y=→"WS1.4":dbl)
      }
    }
    n1550 = case shown="True" "Prog Uno" {
      frame False {
      }
      frame True {
        n1551 = stacked-sequence {
          frame #0 {
            n1552 = Delete(path (use dialog)=path "C:/LAB-IQ-NXT/UNOCOMPILE.bat" ("working directory")) -> ()  [unwired: 4 in, 3 out]
          }
          frame #1 {
            n1553 = local read "Com Port 1"() -> (w1297:refnum<visa-resource-name>)
            n1554 = Concatenate Strings("cmd.exe /c \"mode " ("command line"), w1297, ":1200,n,8,1\"\n" ("command line")) -> (w1302:string)
            n1555 = Concatenate Strings(w1302, "CD\\\nCD WinDucom\navrdude -C avrdude.conf -v -patmega328p -carduino -P" ("command line"), w1297, " -b115200 -D -Uflash:w:UNO_V20.hex:i\n" ("command line"), "\r") -> (w1304:string)
            "STR" <- w1304
            n1556 = call <vilib>:"Write Characters To File.vi"("append to file? (new file:F)"=FALSE, "character string"=w1304, "file path (dialog if empty)"=path "C:/LAB-IQ-NXT/UNOCOMPILE.bat" ("working directory")) -> ()  [unwired: 2 in, 1 out]
          }
          frame #2 {
            n1557 = case shown="True" "Case Constant\n(See Context Help) 10" {
              frame False {
              }
              frame True {
                w1310 = "cmd.exe  /c \"C:\\LAB-IQ-NXT\\UNOCOMPILE.bat\"" ("string")
                n1558 = call <vilib>:"System Exec.vi"("expected output size  (4096)"=u32 65535, "run minimized? (F)"=FALSE, "wait until completion? (T)"=TRUE ("run minimized? (F)"), "working directory"=path "C:/LAB-IQ-NXT", "standard input"=w1310, "command line"=w1310) -> ("error out"=w1309:errorcluster, "standard output"=→"String 42":string)  [unwired: 2 in, 2 out]
                "error out 3" <- w1309
                n1559 = flat-sequence {
                  tunnel: w1309 -> [_]
                  frame #0 {
                  }
                }
              }
            }
            n1560 = local write "Prog Uno"(FALSE ("run minimized? (F)")) -> ()
          }
        }
      }
    }
    n1561 = case shown="True" "Prog Due" {
      frame False {
      }
      frame True {
        n1562 = stacked-sequence {
          frame #0 {
            n1563 = Delete(path (use dialog)=path "C:/LAB-IQ-NXT/DUECOMPILE.bat" ("working directory")) -> ()  [unwired: 4 in, 3 out]
          }
          frame #1 {
            n1564 = case shown="True" "Case Constant\n(See Context Help) 11" {
              frame False {
              }
              frame True {
                n1565 = local read "visa due"() -> (w1278:string)
                n1566 = Concatenate Strings("cmd.exe /c \"mode " ("command line"), w1278, ":1200,n,8,1\"\n" ("command line")) -> (w1283:string)
                n1567 = Concatenate Strings(w1283, "CD\\\nCD WinDucom\nTIMEOUT 1\n bossac.exe -i -d --port=" ("command line"), w1278, " -U false -e -w -v -b DUE.bin -R\n" ("command line"), "\r") -> (w1285:string)
                "concatenated string 2" <- w1285
                n1568 = call <vilib>:"Write Characters To File.vi"("append to file? (new file:F)"=FALSE, "character string"=w1285, "file path (dialog if empty)"=path "C:/LAB-IQ-NXT/DUECOMPILE.bat" ("working directory")) -> ()  [unwired: 2 in, 1 out]
              }
            }
          }
          frame #2 {
            # "C:\\LAB-IQ-NXT\\DUECOMPILE.bat"
            n1569 = case shown="True" "Case Constant\n(See Context Help) 12" {
              frame False {
              }
              frame True {
                w1291 = "cmd.exe  /c \"C:\\LAB-IQ-NXT\\DUECOMPILE.bat\"" ("string")
                n1570 = call <vilib>:"System Exec.vi"("expected output size  (4096)"=u32 65535, "run minimized? (F)"=FALSE, "wait until completion? (T)"=TRUE ("run minimized? (F)"), "working directory"=path "C:/LAB-IQ-NXT", "standard input"=w1291, "command line"=w1291) -> ("error out"=w1290:errorcluster, "standard output"=→"String 44":string)  [unwired: 2 in, 2 out]
                "error out 4" <- w1290
                n1571 = flat-sequence {
                  tunnel: w1290 -> [_]
                  frame #0 {
                  }
                }
              }
            }
            n1572 = local write "Prog Due"(FALSE ("Prog Due")) -> ()
          }
        }
      }
    }
    n1573 = flat-sequence {
      frame #0 {
        n1574 = local read "x = y?"() -> (w1320:bool)
        n1575 = And(x="EDIT", y=w1320) -> (x .and. y?=w1318:bool)
        n1576 = case shown="True" "SAVE" {
          frame False {
          }
          frame True {
            n1577 = stacked-sequence {
              seq-local: [w1521 _ _] -> [_ w1677 _]
              frame #0 {
                (unwired) i16 5 ("precision (6)")
                # "[CH1]    - FF\n[CH2]   - TEMPERATURE\n[CH3]    - Humidity\n[CH4]    - AIR TEMP\n[CH5]\\- Visa Uno\n[CH6] \\- Visa Due\n[CH7]  \\- file path\n[CH8]   - Displacement Gain\n[CHA]   - Stroke Gain\n[CHB]   - Stroke PID Gain\n[CHC]   -Language Selection\n[CHD]   -Power +\n[CHE]   -Power_\n[CHF]   -Heater\n[CHG]   -Humidity Wet\n[CHH]   -Humidity Dry\n[CHI]   -Integral Time"
                n1578 = local read "Com Port 1"() -> (w1512:refnum<visa-resource-name>)
                n1579 = local read "AIR TEMPERATURE :"() -> (w1508:dbl)
                n1580 = local read "DISPLACEMENT :"() -> (w1506:dbl)
                n1581 = local read "HUMIDITY:"() -> (w1507:dbl)
                n1582 = local read "Com Port 2"() -> (w1511:refnum<visa-resource-name>)
                n1583 = local read "TEMPERATURE :"() -> (w1509:dbl)
                n1584 = local read "Stroke PID Gains"() -> (w1572:T9)
                n1585 = local read "FRIC. FORCE :"() -> (w1510:dbl)
                n1586 = local read "STROKE GAIN :"() -> (w1505:dbl)
                n1587 = Unbundle By Name(w1572) -> ("Proportional Gain (Kc)"=w1571:dbl, "Integral Time (Ti, min)"=w1513:dbl)
                n1588 = local read "CH-HUMIDITY DRY"() -> (w1524:u16)
                n1589 = Path To String(path="File Path") -> (string=w1594:string)
                n1590 = local read "Language Selection"() -> (w1569:enum16{"English", "Russian"})
                n1591 = local read "CH-POWER +"() -> (w1536:u16)
                n1592 = local read "CH-HUMIDITY WET"() -> (w1527:u16)
                n1593 = Number To Fractional String(number=w1507, width (-)=i16 10 ("precision (6)"), precision (6)=i16 5) -> (F-format string=w1619:string)  [unwired: 1 in]
                n1594 = Concatenate Strings(w1594, "\\" ("string")) -> (w1593:string)
                n1595 = local read "CH-POWER -"() -> (w1533:u16)
                n1596 = Number To Fractional String(number=w1509, width (-)=i16 10 ("precision (6)"), precision (6)=i16 5) -> (F-format string=w1625:string)  [unwired: 1 in]
                n1597 = Number To Fractional String(number=w1508, width (-)=i16 10 ("precision (6)"), precision (6)=i16 5) -> (F-format string=w1613:string)  [unwired: 1 in]
                n1598 = Number To Fractional String(number=w1506, width (-)=i16 10 ("precision (6)"), precision (6)=i16 5) -> (F-format string=w1586:string)  [unwired: 1 in]
                n1599 = local read "CH-HEATER"() -> (w1530:u16)
                n1600 = Number To Fractional String(number=w1505, width (-)=i16 10 ("precision (6)"), precision (6)=i16 5) -> (F-format string=w1585:string)  [unwired: 1 in]
                n1601 = Number To Fractional String(number=w1510, width (-)=i16 10 ("precision (6)"), precision (6)=i16 5) -> (F-format string=w1626:string)  [unwired: 1 in]
                n1602 = Number To Fractional String(number=w1571, width (-)=i16 10 ("precision (6)"), precision (6)=i16 5) -> (F-format string=w1573:string)  [unwired: 1 in]
                n1603 = Number To Fractional String(number=w1569, width (-)=i16 10 ("precision (6)"), precision (6)=i16 5) -> (F-format string=w1565:string)  [unwired: 1 in]
                n1604 = Number To Fractional String(number=w1536, width (-)=i16 10 ("precision (6)"), precision (6)=i16 5) -> (F-format string=w1559:string)  [unwired: 1 in]
                n1605 = Number To Fractional String(number=w1533, width (-)=i16 10 ("precision (6)"), precision (6)=i16 5) -> (F-format string=w1556:string)  [unwired: 1 in]
                n1606 = Number To Fractional String(number=w1530, width (-)=i16 10 ("precision (6)"), precision (6)=i16 5) -> (F-format string=w1551:string)  [unwired: 1 in]
                n1607 = Number To Fractional String(number=w1527, width (-)=i16 10 ("precision (6)"), precision (6)=i16 5) -> (F-format string=w1548:string)  [unwired: 1 in]
                n1608 = Number To Fractional String(number=w1524, width (-)=i16 10 ("precision (6)"), precision (6)=i16 5) -> (F-format string=w1543:string)  [unwired: 1 in]
                n1609 = Concatenate Strings("[CH1]" ("string"), w1626, " - FF" ("string"), "\r") -> (w1624:string)
                n1610 = Concatenate Strings("[CH3]" ("string"), w1619, " - Humidity" ("string"), "\r") -> (w1616:string)
                n1611 = Concatenate Strings("[CH7]" ("string"), w1593, "- file path" ("string"), "\r") -> (w1596:string)
                n1612 = Number To Fractional String(number=w1513, width (-)=i16 10 ("precision (6)"), precision (6)=i16 5) -> (F-format string=w1517:string)  [unwired: 1 in]
                n1613 = Concatenate Strings("[CH6]" ("string"), w1511, "- Visa Due" ("string"), "\r") -> (w1597:string)
                n1614 = Concatenate Strings("[CH8]" ("string"), w1586, "- Displacement Gain" ("string"), "\r") -> (w1589:string)
                n1615 = Concatenate Strings("[CHA]" ("string"), w1585, "- Stroke Gain" ("string"), "\r") -> (w1579:string)
                n1616 = Concatenate Strings("[CH5]" ("string"), w1512, "- Visa Uno" ("string"), "\r") -> (w1602:string)
                n1617 = Concatenate Strings("[CH4]" ("string"), w1613, " - AIR TEMP" ("string"), "\r") -> (w1609:string)
                n1618 = Concatenate Strings("[CH2]" ("string"), w1625, " - TEMPERATURE" ("string"), "\r") -> (w1623:string)
                n1619 = Concatenate Strings("[CHC]" ("string"), w1565, "-Language Selection" ("string"), "\r") -> (w1562:string)
                n1620 = Concatenate Strings("[CHD]" ("string"), w1559, "-Power +" ("string"), "\r") -> (w1541:string)
                n1621 = Concatenate Strings("[CHE]" ("string"), w1556, "-Power_" ("string"), "\r") -> (w1540:string)
                n1622 = Concatenate Strings("[CHF]" ("string"), w1551, "-Heater" ("string"), "\r") -> (w1539:string)
                n1623 = Concatenate Strings("[CHB]" ("string"), w1573, "- Stroke PID Gain" ("string"), "\r") -> (w1570:string)
                n1624 = Concatenate Strings("[CHG]" ("string"), w1548, "-Humidity Wet" ("string"), "\r") -> (w1538:string)
                n1625 = Concatenate Strings("[CHH]" ("string"), w1543, "-Humidity Dry" ("string"), "\r") -> (w1537:string)
                n1626 = Concatenate Strings("[CHI]" ("string"), w1517, "-Integral Time " ("string"), "\r") -> (w1514:string)
                n1627 = Concatenate Strings(w1624, w1623, w1616, w1609, w1602, w1597, w1596, w1589, w1579, w1570, w1562, w1541, w1540, w1539, w1538, w1537, w1514) -> (w1521:string)
                "gain" <- w1521
              }
              frame #1 {
                n1628 = local read "AIR TEMP INTERCEPT:"() -> (w1638:dbl)
                n1629 = local read "TEMP INTERCEPT:"() -> (w1637:dbl)
                n1630 = local read "Com Port 3"() -> (w1647:refnum<visa-resource-name>)
                n1631 = local read "LvdtOff"() -> (w1640:dbl)
                n1632 = Number To Fractional String(number=w1637, width (-)=i16 10 ("precision (6)"), precision (6)=i16 5) -> (F-format string=w1665:string)  [unwired: 1 in]
                n1633 = Number To Fractional String(number=w1638, width (-)=i16 10 ("precision (6)"), precision (6)=i16 5) -> (F-format string=w1672:string)  [unwired: 1 in]
                n1634 = Number To Fractional String(number=w1640, width (-)=i16 10 ("precision (6)"), precision (6)=i16 5) -> (F-format string=w1644:string)  [unwired: 1 in]
                n1635 = Concatenate Strings("[CHK]" ("string"), w1665, "-TEMP INTERCEPT" ("string"), "\r") -> (w1661:string)
                n1636 = Concatenate Strings("[CHJ]" ("string"), w1672, "-AIR TEMP INTERCEPT" ("string"), "\r") -> (w1662:string)
                n1637 = Concatenate Strings("[SNO]" ("string"), "S.NO", "-" ("string"), "\r") -> (w1657:string)
                n1638 = Concatenate Strings("[CHL]" ("string"), w1647, "- Visa humid" ("string"), "\r") -> (w1650:string)
                n1639 = Concatenate Strings("[CHI]" ("string"), w1644, "-LVDT Position Offset" ("string"), "\r") -> (w1639:string)
                n1640 = Concatenate Strings(w1677, w1662, w1661, w1657, w1650, w1639) -> (w1676:string)
                n1641 = local read "Gain path"() -> (w1655:string)
                n1642 = Concatenate Strings(w1655, "\\calibrate std ED hfrr.dcf") -> ()  [unwired: 1 out]
                n1643 = String To Path(string="C:\\LAB-IQ-NXT\\calibrate WO 2464.dcf") -> (path=w1648:path)
                n1644 = call <vilib>:"Write Characters To File.vi"("append to file? (new file:F)"=FALSE, "character string"=w1676, "file path (dialog if empty)"=w1648) -> ()  [unwired: 2 in, 1 out]
              }
              frame #2 {
                n1645 = local write "Lan flag"(0.0 ("Lan flag")) -> ()
                n1646 = local write "Re-Initialise"(TRUE ("Re-Initialise")) -> ()
                n1647 = local write "conststatus"(0.0 ("rpm value : 2")) -> ()
                n1648 = local write "SAVE"(FALSE ("OK Button 14")) -> ()
              }
            }
          }
        }
        n1649 = case shown="False" w1318 {
          tunnel: [u8 2 ("Disabled") u8 0 ("Disabled")] -> w1317
          tunnel: [w1682 TRUE ("Visible")] -> w1316
          frame False {
            w1682 = FALSE ("Visible")
            n1650 = local write "EDIT 2"(w1682) -> ()
          }
          frame True {
          }
        }
        n1651 = property on="Tab Control" class="TabCtl (strict)"("Visible"=w1316) -> ()  [unwired: 2 in, 2 out]
        n1652 = property on="EDIT 2" class="Bool (strict)"("Visible"=w1316) -> ()  [unwired: 2 in, 2 out]
        n1653 = property on="TEMPERATURE :" class="DigNum (strict)"("Disabled"=w1317) -> ()  [unwired: 2 in, 2 out]
        n1654 = property on="SAVE" class="Bool (strict)"("Visible"=w1316) -> ()  [unwired: 2 in, 2 out]
        n1655 = property on="AIR TEMPERATURE :" class="DigNum (strict)"("Disabled"=w1317) -> ()  [unwired: 2 in, 2 out]
        n1656 = property on="SPEED OUT:" class="DigNum (strict)"("Disabled"=w1317) -> ()  [unwired: 2 in, 2 out]
        n1657 = property on="HUMIDITY:" class="DigNum (strict)"("Disabled"=w1317) -> ()  [unwired: 2 in, 2 out]
        n1658 = property on="FRIC. FORCE :" class="DigNum (strict)"("Disabled"=w1317) -> ()  [unwired: 2 in, 2 out]
        n1659 = property on="Tab Control 7" class="TabCtl (strict)"("Disabled"=w1317) -> ()  [unwired: 2 in, 2 out]
